vi "CV.vi"(1 "Wait for continue":bool, 2 "Run uninterrupted?":bool, 3 "Device Category IN:":string(combo)="ATLAS18SS" caption="Device Category:", 4 "Batch :":string, 5 "Wafer No.:":string, 6 "DB Serial No.:":string) -> (0 "Done!":bool=TRUE)   [LabVIEW 2018]
doc: "Performs CV measurements according to ATLAS ITk Quality Control Specifications."
uses:
  general_VIs/globals/QC_MeasurementSetup.vi
  general_VIs/globals/QC_RunInformation.vi
  InstrControl/InstrumentSetup.vi
  InstrControl/Switching/Switching.lvclass
  InstrControl/SupplyControl/SupplyControl.lvclass
  InstrControl/LCRControl/LCRControl.lvclass
  InstrControl/ArduinoControl/ArduinoControl.lvclass
  InstrControl/InstrControl.lvclass
panel:
  out "Tab Control 2":enum32{"CV Setup", "CV Scan"}(tab)
  in  "V_depletion limit [V]":dbl=-300.0
  in  "step interval [s] IN":i32=5 caption="step interval [s]"
  in  "step [V] IN":dbl=10.0 caption="step [V]" format="%.1f"
  in  "Final volts [V] IN":dbl=-700.0 caption="Final volts [V]"
  in  "Initial volts [V] IN":dbl caption="Initial volts [V]"
  in  "Current Limit [µA]":dbl=1.0 min=0.0001 format="%.3f"
  in  "Continue":bool
  in  "Quit":bool
  in  "Software current limit?":bool=TRUE
  out "Frequency [Hz] Setup":i32=1000 caption="Frequency [Hz]" format="%#.3p"
  in  "Measurement Configurations":bool
  out "RH":dbl[](array[numeric])=[8.13] caption="RH [%]" format="%#.2f"
  out "step interval [s]":u32=5
  out "step [V]":dbl=10.0 format="%.1f"
  out "Final volts [V]":dbl=-500.0 format="%.1f"
  out "Initial volts [V]":dbl format="%.1f"
  out "Frequency [Hz]":i32=1000 format="%#.3p"
  out "Temp.":dbl[](array[numeric])=[22.58] caption="Temp. [°C]" format="%#.2f"
  out "Volts":dbl[](array[numeric])=[-460.0, -470.0, -480.0, -490.0, -500.0] caption="Volts [V]"
  out "Resistance":dbl[](array[numeric])=[1.56271, 1.56475, 1.51322, 1.51532, 1.51442] caption="Res [kOhm]"
  out "Capacitance":dbl[](array[numeric])=[3119.33, 3118.74, 3118.2400000000002, 3117.68, 3117.2799999999997] caption="Cap [pF]"
  out "Cgraph":cluster{"Initial volts":dbl, dbl, dbl[]}(graph)={"Initial volts"=0.0, 10.0, [5.7235032491421625e-05, 0.003217145788776149, 0.00672998297054733, 0.010666134294020897, 0.014929833398235195, 0.018713223783299704, 0.022188100626603195, 0.025608357885954832, 0.028957991168771992, 0.03227724289159167, 0.03580683190419423, 0.03921028907816598, 0.04253563831220547, 0.045835956575624094, 0.04914718334784051, 0.0524545061658223, 0.055801253982253135, 0.05918861335467005, 0.06262205347418506, 0.06605343343205772, 0.06951342144191594, 0.0730175985670206, 0.07657909511703177, 0.0802264781180157, 0.08403593560473727, 0.08800309677997556, 0.09205485037916886, 0.09598073570407974, 0.09910778032065119, 0.10069600303043066, 0.10132328993192792, 0.1016323293588705, 0.10182246094227795, 0.10197208503414133, 0.10207832275216988, 0.10217166194307145, 0.10225008736408765, 0.1023214020753015, 0.10238361796587031, 0.10244457903006766, 0.10248262532843988, 0.10253579443044537, 0.10258769058231139, 0.10262976192794523, 0.10266988527288097, 0.1027152990629271, 0.10277260288908789, 0.10281149139612399, 0.10284446503963636, 0.10288141435634753, 0.10290781891803549]}
  in  "Scales":T1(ring)
  in  "Cscale":enum16{"1/C^2 [1/nF^2]", "nF", "pF"}(ring)
  out "positive ramp?":bool
  out "Tab Control":enum32{"CV Setup", "CV Scan"}(tab)
  in  "Comments":string caption="Comments:"
  in  "Auto save files":bool=TRUE
  in  "LCR Meter":string(combo)="HP 4284A"
  in  "User:":string(combo)="Vera"
  in  "CV Supply":string(combo)="Keithley 237"
  in  "Hardware Configurations":bool
  in  "Temperature":enum16{"Read Arduino", "Enter manually"}(ring)
  in  "Manufacturer:":string(combo)="Hamamatsu"
  in  "abort":bool
  out "Device Category:":string="ATLAS18SS"
  out "DB Serial No.:":string="20USES50000070"
  out "Current Volts:":dbl format="%.2f"
  in  "quit (no save)":bool
  in  "Quit & Save":bool
  out "Bias On/Off:":bool
  out "STATUS 1":string="Run finished.\nData saved."
  out "Initiated:":string="Thu, Jul 9, 2020"
  out "Wafer:":string="W070"
  out "No of steps":u32=71
  out "Current reading No.":u32=51
  out "Last reading at:":string="2:43:44 PM"
  # "Strip Sensor QC: CV"
  # "University of\nCambridge"
  # "Vertical Scale:"
  # "Measurement Configuration"
  # "CV Scan parameters:"
  # "Last 5 readings:"
  # "n-4"
  # "n-3"
  # "n-2"
  # "n-1"
  # "n"
  # "DUT Description"
  # "Hardware"
  # "DUT & Test Description:"
  # "Current status:"
  # "Rdg No:"
  # "out of"
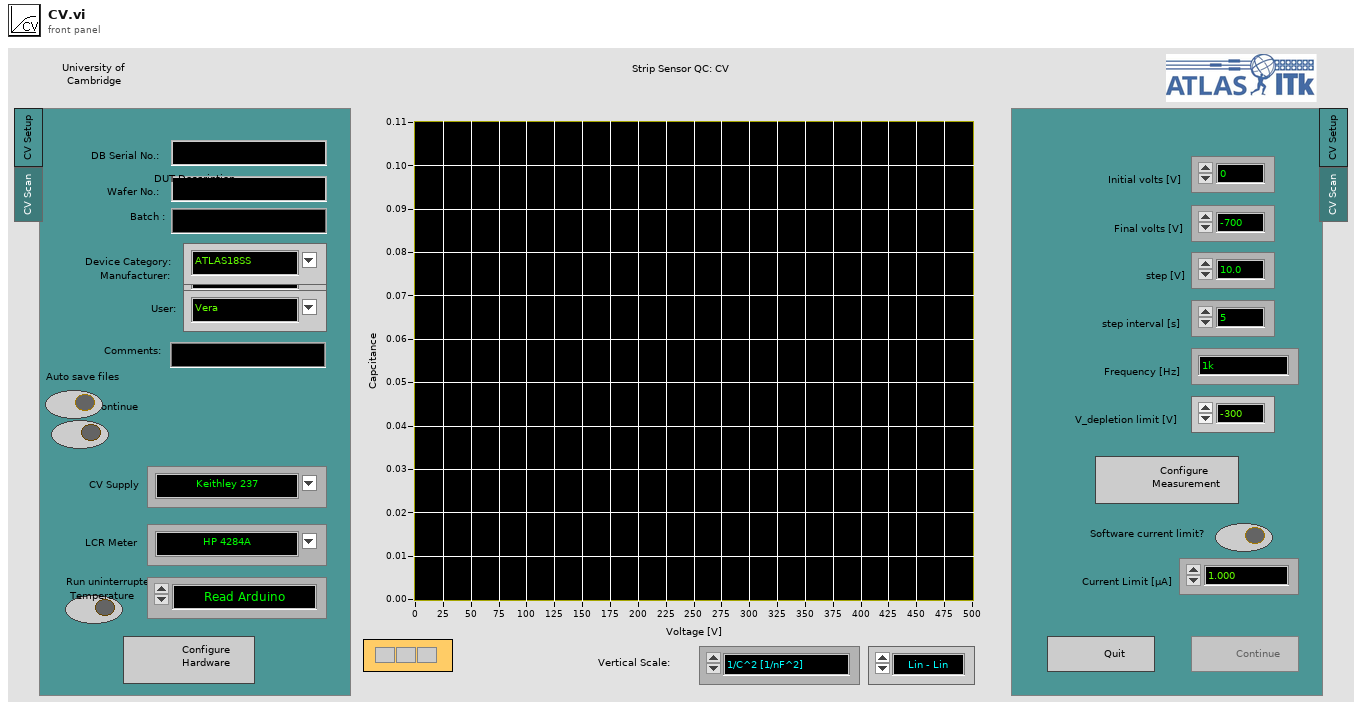
[diagram p1: front panel]
types:
  T1 = enum16{"Lin - Lin", "Log - Lin", "Lin - Log", "Log - log"}
  T2 = enum16{"Supply", "LCR", "Multimeter", "Switching"}
  T3 = enum16{"Reset", "Read Array", "Read Element", "Write Element", "Write Array", "Add Element", "Add Array"}
  T4 = enum16{"Reset", "Ground", "Striptest SMU", "Striptest LCR", "IV", "CV", "Interstrip Cap", "Interstrip Res"}
  T5 = enum32{"IV", "CV", "Stability", "Striptest", "Cis", "Ris", "PTP"}
  T6 = cluster{"Sensor Serial No.:":string, "Wafer:":string, "Batch:":string, "Manufacturer:":string, "Device Category:":string, "Database Serial No.:":string, "Date Initiated:":string, "Time Initiated:":string, "Test":string, "Probeplan used:":string, "End of Run comment:":string, "User:":string, "Vbias SMU":string, "LCR":string, "Test SMU":string, "Test DMM":string, "Comments":string}
  T7 = cluster{"Institute":string, "Manufacturers":string[], "Devices":string[], "Serialnumbers Lookup DB":string, "Data directory":string, "Backup & screenshot directory":string, "List of known users":string[], "Measurement switch not used":bool, "Measurement Switch":string, "DUT Switch":string, "Rseries IV [MOhm]":string, "Rshunt IV [MOhm]":string, "Rseries CV [MOhm]":string, "DC blocking Cap [µF]":string, "Rseries LCR [MOhm]":string, "Rseries stability [MOhm]":string, "Rshunt stability [MOhm]":string, "Rseries striptest bias [MOhm]":string, "Rseries strip pinhole [MOhm]":string}
  T8 = cluster{"Supply":refnum<class "SupplyControl.lvclass">, "LCR":refnum<class "LCRControl.lvclass">, "Arduino":refnum<class "ArduinoControl.lvclass">, "Measurement switch":refnum<class "Switching.lvclass">, "Initial Voltage [V]":dbl, "Final Voltage [V]":dbl, "Step Size [V]":dbl, "Step Interval [s]":i32, "Number Of Steps":u32, "AC frequency [Hz]":i32, "RC Configuration":u16, "AC amplitude [V]":dbl, "Ramp down steps [V]":dbl, "Ramp down Interval [s]":i32, "Set Current Limit?":bool, "Current Limit [µA]":dbl, "Temperature Readout":enum16{"Read Arduino", "Enter manually"}, "Supply Name":string, "LCR Name":string, "V_depletion Limit [V]":dbl, "Measurement switch used?":bool}
  T9 = cluster{"RC Configuration":u16, "AC amplitude [V]":dbl, "Consider OC":bool, "Consider SC":bool, "AC frequency [Hz]":i32, "HP4284A":refnum<class "HP4284A.lvclass">}
  T10 = cluster{"VISA address":refnum<visa-resource-name>, "T sensor":enum16{"SHT", "DS"}, "Arduino":refnum<class "ArduinoControl.lvclass">}
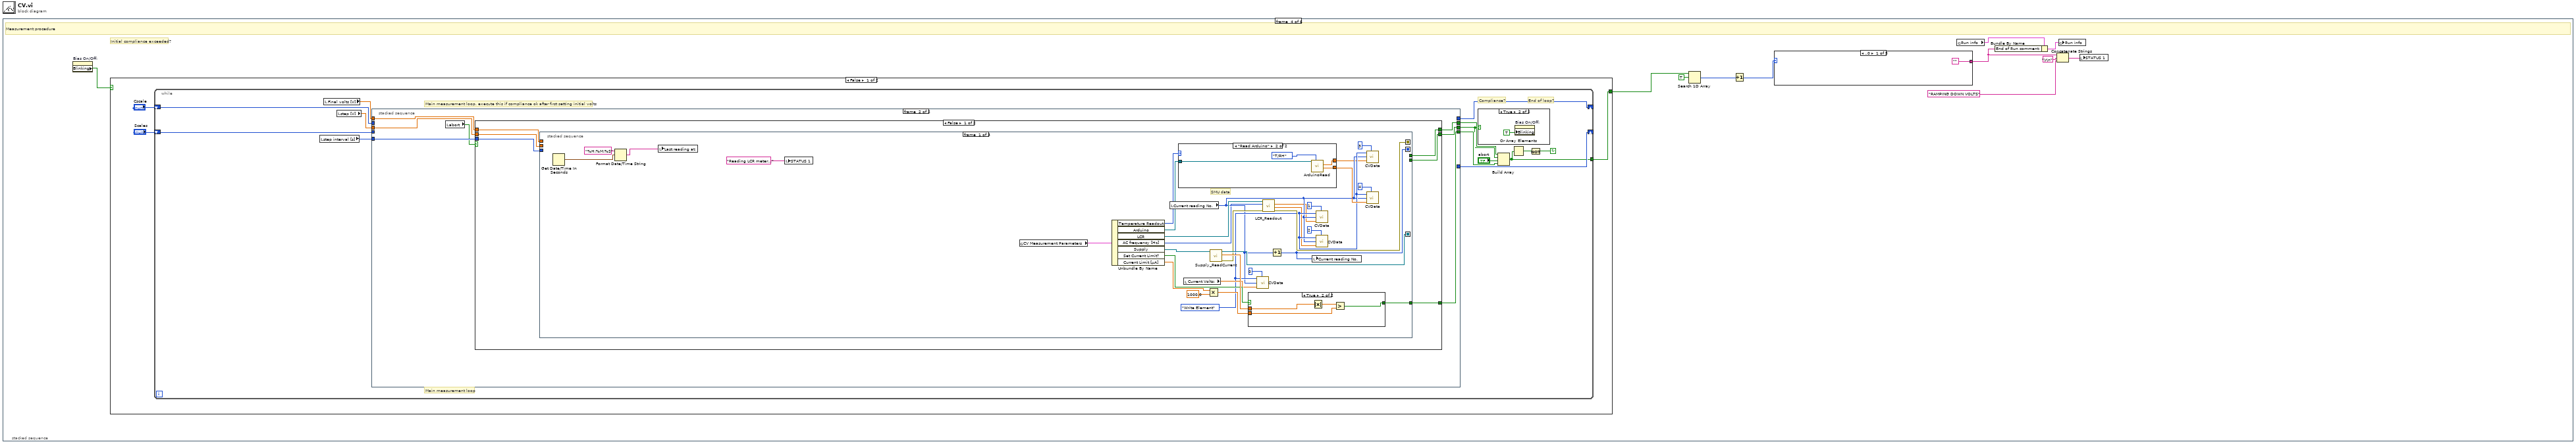
[diagram p0: block diagram]
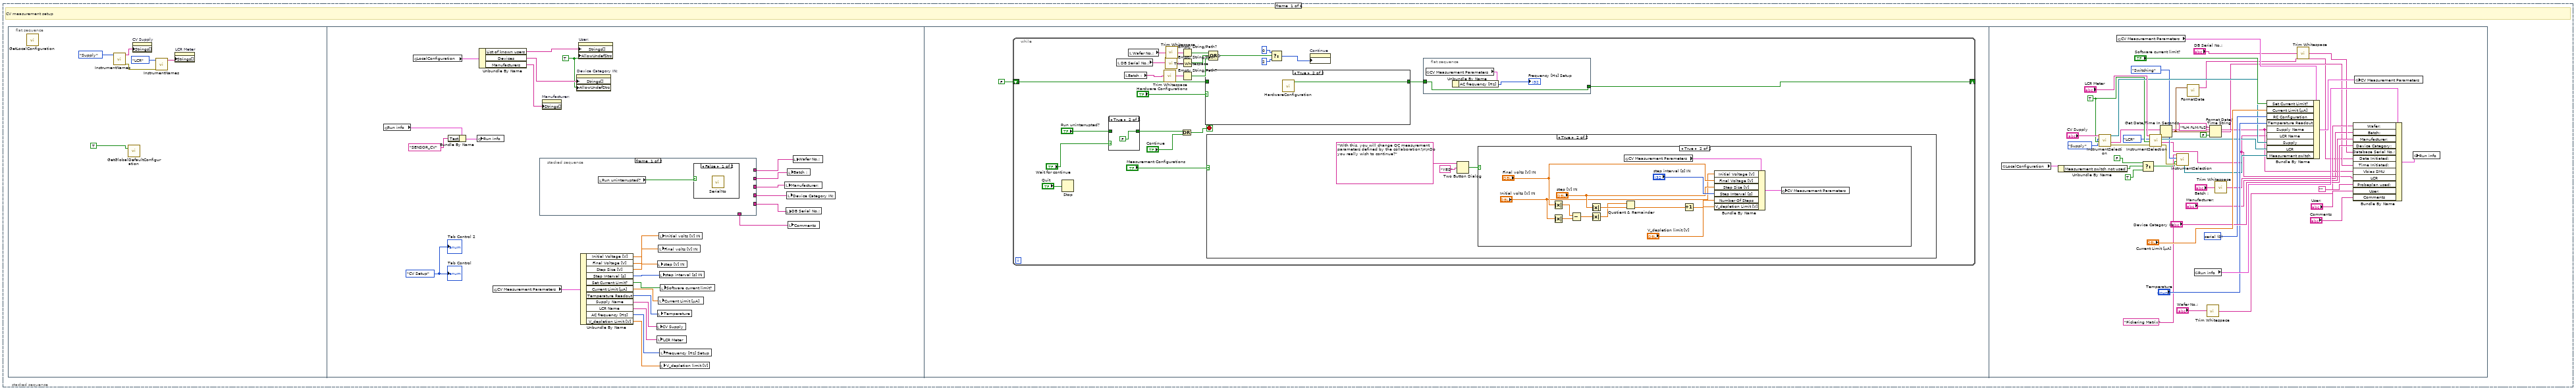
[diagram p2: hidden frame]
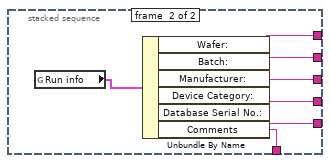
[diagram p4: hidden frame]
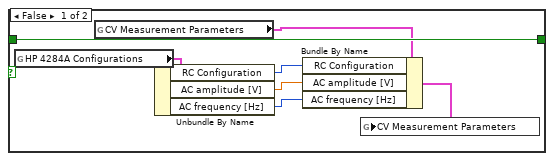
[diagram p6: hidden frame]
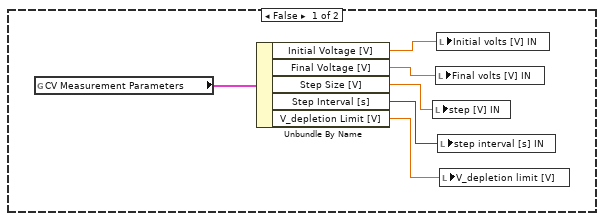
[diagram p8: hidden frame]
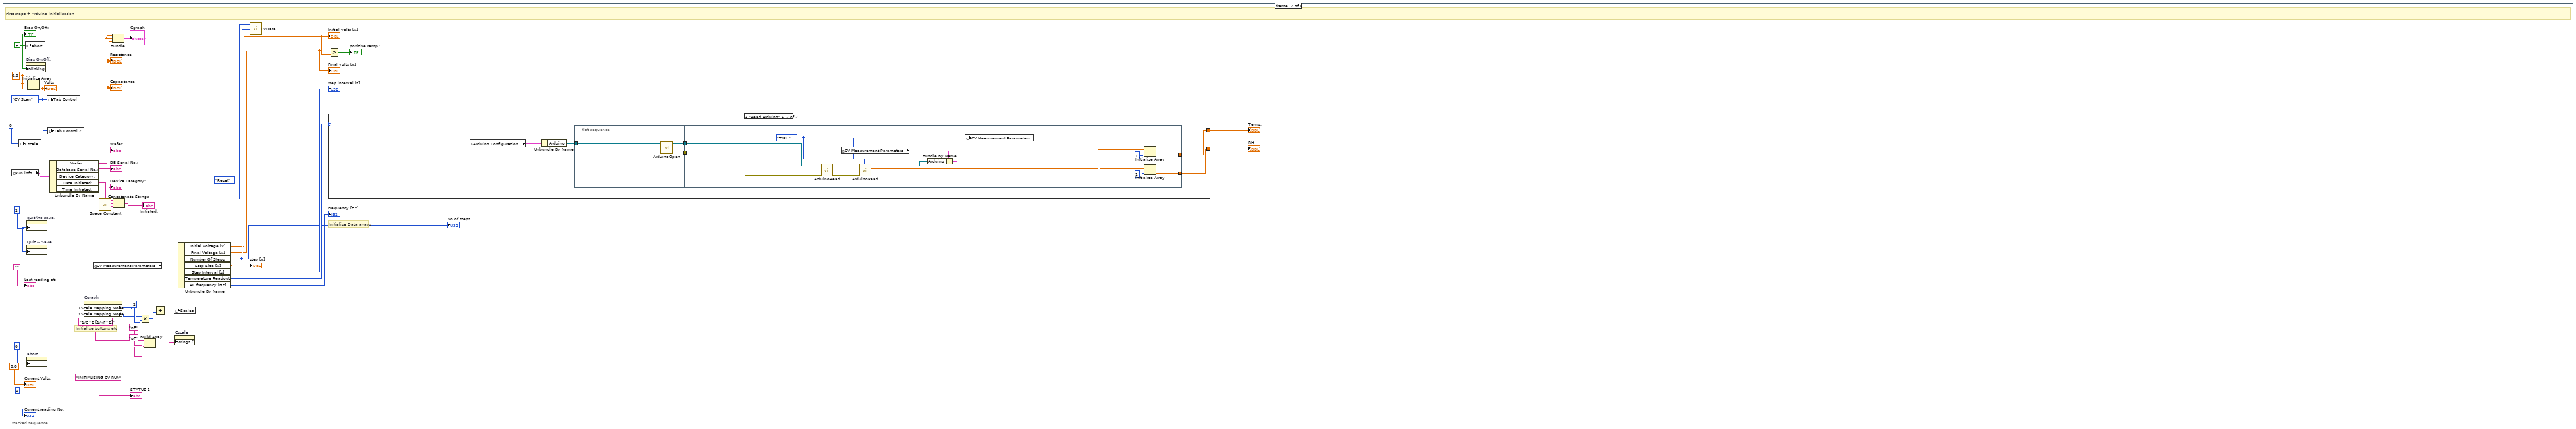
[diagram p9: hidden frame]
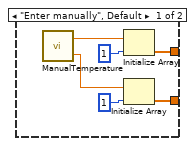
[diagram p10: hidden frame]
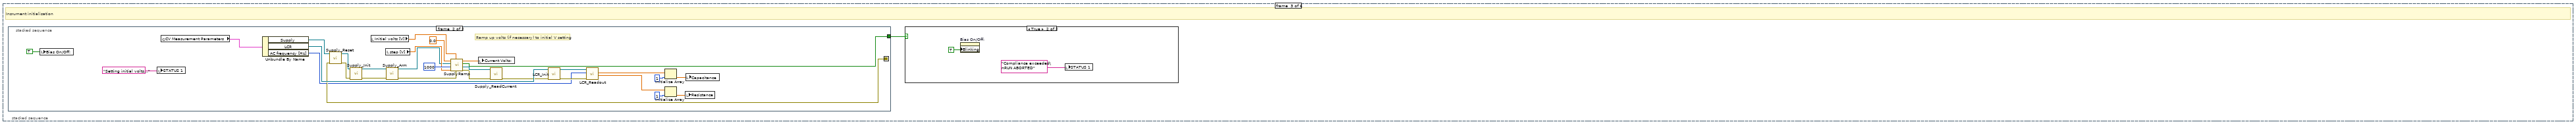
[diagram p11: hidden frame]
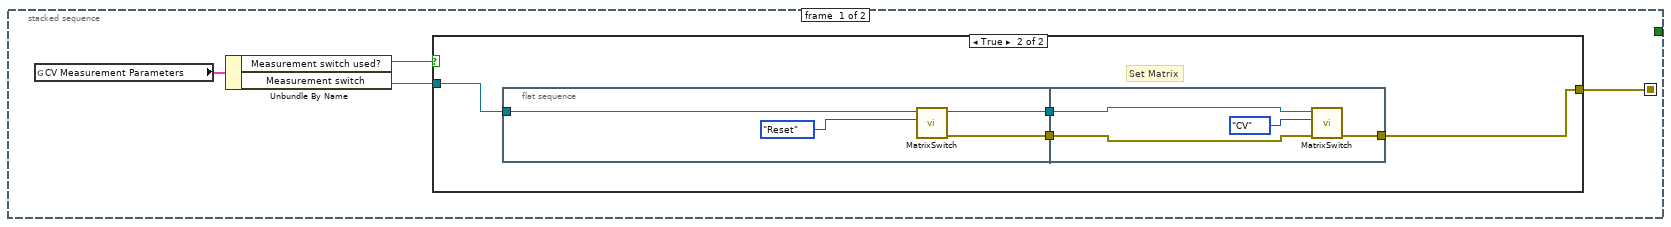
[diagram p12: hidden frame]
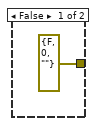
[diagram p13: hidden frame]
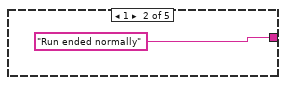
[diagram p15: hidden frame]
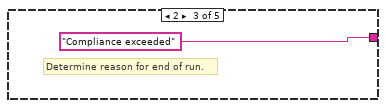
[diagram p16: hidden frame]
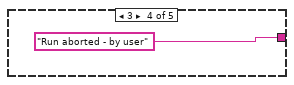
[diagram p17: hidden frame]
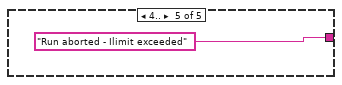
[diagram p18: hidden frame]
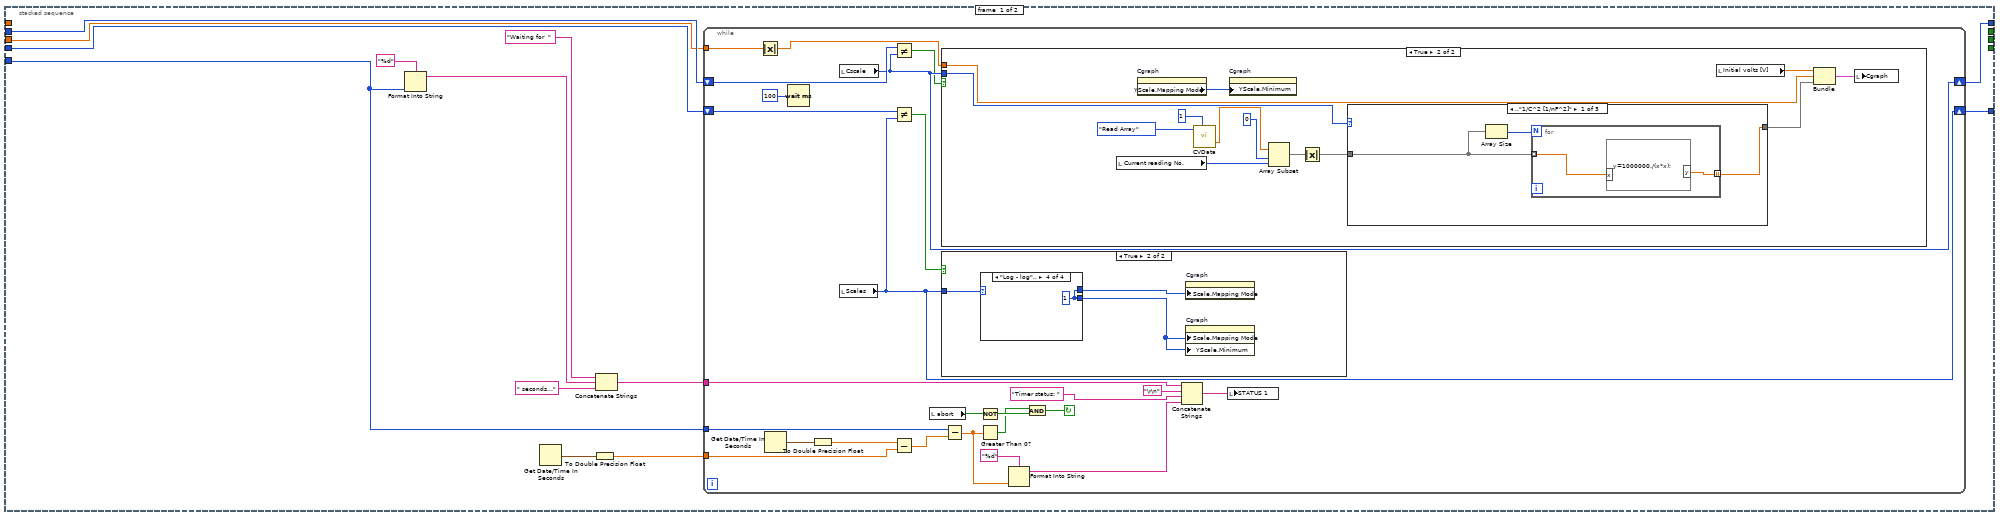
[diagram p19: hidden frame]
diagram:
  n1 = stacked-sequence {
    frame #0 {
      # "CV measurement setup"
      n2 = flat-sequence {
        frame #0 {
          n3 = call "GetLocalConfiguration.vi"() -> ()  [unwired: 3 in, 1 out]
          n4 = call "InstrumentNames.vi"("Instrument type"=T2."Supply") -> ("error out"=w1:errorcluster, "Instrument names"=w3:string[])  [unwired: 9 in]
          n5 = call "GetGlobalDefaultConfiguration.vi"("Read defaults?"=TRUE) -> ()  [unwired: 3 in]
          n6 = property on="CV Supply" class="CmbBox"("Strings[]"=w3) -> ()  [unwired: 2 in, 2 out]
          n7 = call "InstrumentNames.vi"("error in (no error)"=w1, "Instrument type"=T2."LCR") -> ("Instrument names"=w2:string[])  [unwired: 8 in, 1 out]
          n8 = property on="LCR Meter" class="CmbBox"("Strings[]"=w2) -> ()  [unwired: 2 in, 2 out]
        }
        frame #1 {
          w22 = enum32{"CV Setup", "CV Scan"}."CV Setup" ("Tab Control")
          w14 = TRUE
          n9 = global read "QC_RunInformation.vi" "Run info"() -> (w23:T6)
          n10 = global read "QC_RunInformation.vi" "LocalConfiguration"() -> (w28:T7)
          n11 = Bundle By Name(cluster=w23, "Test"="SENSOR_CV") -> (w24:T6)
          n12 = global write "QC_RunInformation.vi" "Run info"(w24) -> ()
          n13 = Unbundle By Name(w28) -> ("List of known users"=w27:string[], "Devices"=w15:string[], "Manufacturers"=w16:string[])
          n14 = global read "QC_MeasurementSetup.vi" "CV Measurement Parameters"() -> (w31:T8)
          n15 = stacked-sequence {
            tunnel: [_ w41] -> w12
            tunnel: [_ w40] -> w11
            tunnel: [_ w39] -> w10
            tunnel: [_ w38] -> w13
            tunnel: [_ w36] -> w9
            tunnel: [_ w35] -> w7
            frame #0 {
              n16 = local read "Run uninterrupted?"() -> (w34:bool)
              n17 = case shown="False" w34 {
                frame False {
                  n18 = call "SerialNo.vi"() -> ()  [unwired: 5 in, 1 out]
                }
                frame True {
                }
              }
            }
            frame #1 {
              n19 = global read "QC_RunInformation.vi" "Run info"() -> (w37:T6)
              n20 = Unbundle By Name(w37) -> ("Wafer:"=w41:string, "Batch:"=w40:string, "Manufacturer:"=w39:string, "Device Category:"=w38:string, "Database Serial No.:"=w36:string, "Comments"=w35:string)
            }
          }
          n21 = property on="Manufacturer:" class="CmbBox"("Strings[]"=w16) -> ()  [unwired: 2 in, 2 out]
          n22 = property on="Device Category IN:" class="CmbBox"("Strings[]"=w15, "AllowUndefStrs"=w14) -> ()  [unwired: 2 in, 2 out]
          n23 = property on="User:" class="CmbBox"("Strings[]"=w27, "AllowUndefStrs"=w14) -> ()  [unwired: 2 in, 2 out]
          n24 = Unbundle By Name(w31) -> ("Initial Voltage [V]"=w18:dbl, "Final Voltage [V]"=w19:dbl, "Step Size [V]"=w20:dbl, "Step Interval [s]"=w21:i32, "Set Current Limit?"=w30:bool, "Current Limit [µA]"=w29:dbl, "Temperature Readout"=w33:enum16{"Read Arduino", "Enter manually"}, "Supply Name"=w32:string, "LCR Name"=w26:string, "AC frequency [Hz]"=w25:i32, "V_depletion Limit [V]"=w17:dbl)
          n25 = local write "CV Supply"(w32) -> ()
          n26 = local write "LCR Meter"(w26) -> ()
          n27 = local write "step [V] IN"(w20) -> ()
          n28 = local write "Temperature"(w33) -> ()
          n29 = local write "Final volts [V] IN"(w19) -> ()
          n30 = local write "Current Limit [µA]"(w29) -> ()
          n31 = local write "Initial volts [V] IN"(w18) -> ()
          n32 = local write "step interval [s] IN"(w21) -> ()
          n33 = local write "Frequency [Hz] Setup"(w25) -> ()
          n34 = local write "V_depletion limit [V]"(w17) -> ()
          n35 = local write "Software current limit?"(w30) -> ()
          n36 = local write "Manufacturer:"(w10) -> ()
          n37 = local write "DB Serial No.:"(w9) -> ()
          n38 = local write "Device Category IN:"(w13) -> ()
          n39 = local write "Batch :"(w11) -> ()
          n40 = local write "Comments"(w7) -> ()
          n41 = local write "Wafer No.:"(w12) -> ()
          "Tab Control" <- w22
          "Tab Control 2" <- w22
        }
        frame #2 {
          n42 = while {
            shift-right: [w43] -> _
            shift-left: FALSE -> [w55]
            stop <- w57 stop-if-true
            n43 = Stop(stop? (T)="Quit") -> ()
            n44 = case shown="True" "Wait for continue" {
              tunnel: "Run uninterrupted?" -> [w70 _]
              tunnel: [w70 FALSE] -> w51
              frame False {
              }
              frame True {
              }
            }
            n45 = local read "DB Serial No.:"() -> (w48:string)
            n46 = local read "Batch :"() -> (w46:string)
            n47 = local read "Wafer No.:"() -> (w49:string)
            n48 = call <vilib>:"Trim Whitespace.vi"("string"=w46) -> ("trimmed string"=w45:string)  [unwired: 1 in]
            n49 = call <vilib>:"Trim Whitespace.vi"("string"=w48) -> ("trimmed string"=w47:string)  [unwired: 1 in]
            n50 = call <vilib>:"Trim Whitespace.vi"("string"=w49) -> ("trimmed string"=w50:string)  [unwired: 1 in]
            n51 = Or(x=w51, y="Continue") -> (x .or. y?=w57:bool)
            n52 = Empty String/Path?(string/path=w50) -> (empty?=w64:bool)
            n53 = Empty String/Path?(string/path=w47) -> (empty?=w65:bool)
            n54 = Empty String/Path?(string/path=w45) -> (empty?=w59:bool)
            n55 = case shown="True" "Hardware Configurations" {
              tunnel: [w78 w79] -> w44
              tunnel: w55 -> [w78 _]
              frame False {
                n56 = global read "InstrumentSetup.vi" "HP 4284A Configurations"() -> (w77:T9)
                n57 = global read "QC_MeasurementSetup.vi" "CV Measurement Parameters"() -> (w76:T8)
                n58 = Unbundle By Name(w77) -> ("RC Configuration"=w75:u16, "AC amplitude [V]"=w74:dbl, "AC frequency [Hz]"=w73:i32)
                n59 = Bundle By Name(cluster=w76, "RC Configuration"=w75, "AC amplitude [V]"=w74, "AC frequency [Hz]"=w73) -> (w72:T8)
                n60 = global write "QC_MeasurementSetup.vi" "CV Measurement Parameters"(w72) -> ()
              }
              frame True {
                n61 = call "HardwareConfiguration.vi"() -> ("configured?"=w79:bool)  [unwired: 11 in]
              }
            }
            n62 = case shown="True" "Measurement Configurations" {
              frame False {
              }
              frame True {
                n63 = Two Button Dialog(message="With this, you will change QC measurement parameters defined by the collaboration!\n\nDo you really wish to continue?", 2:"YES") -> (T button?=w80:bool)  [unwired: 1 in]
                n64 = case shown="True" w80 {
                  frame False {
                    n65 = global read "QC_MeasurementSetup.vi" "CV Measurement Parameters"() -> (w88:T8)
                    n66 = Unbundle By Name(w88) -> ("Initial Voltage [V]"=w85:dbl, "Final Voltage [V]"=w84:dbl, "Step Size [V]"=w86:dbl, "Step Interval [s]"=w87:i32, "V_depletion Limit [V]"=w83:dbl)
                    n67 = local write "step [V] IN"(w86) -> ()
                    n68 = local write "Final volts [V] IN"(w84) -> ()
                    n69 = local write "Initial volts [V] IN"(w85) -> ()
                    n70 = local write "step interval [s] IN"(w87) -> ()
                    n71 = local write "V_depletion limit [V]"(w83) -> ()
                  }
                  frame True {
                    n72 = Absolute Value(x="Final volts [V] IN") -> (abs(x)=w94:dbl)
                    n73 = Absolute Value(x="Initial volts [V] IN") -> (abs(x)=w95:dbl)
                    n74 = Subtract(x=w94, y=w95) -> (x-y=w98:dbl)
                    n75 = Absolute Value(x="step [V] IN") -> (abs(x)=w97:dbl)
                    n76 = Absolute Value(x=w98) -> (abs(x)=w96:dbl)
                    n77 = global read "QC_MeasurementSetup.vi" "CV Measurement Parameters"() -> (w102:T8)
                    n78 = Quotient & Remainder(x=w96, y=w97) -> (floor(x/y)=w93:dbl)  [unwired: 1 out]
                    n79 = Increment(x=w93) -> (x+1=w92:dbl)
                    n80 = Bundle By Name(cluster=w102, "Initial Voltage [V]"="Initial volts [V] IN", "Final Voltage [V]"="Final volts [V] IN", "Step Size [V]"="step [V] IN", "Step Interval [s]"="step interval [s] IN", "Number Of Steps"=w92, "V_depletion Limit [V]"="V_depletion limit [V]") -> (w101:T8)
                    n81 = global write "QC_MeasurementSetup.vi" "CV Measurement Parameters"(w101) -> ()
                  }
                }
              }
            }
            n82 = Compound Arithmetic op=OR(w64, w65, w59) -> (invert w63:bool)
            n83 = Select(t=0, s=w63, f=2) -> (s? t:f=w60:i32)
            n84 = property on="Continue" class="Bool"("DisabledEnum"=w60) -> ()  [unwired: 2 in, 2 out]
            n85 = flat-sequence {
              tunnel: w44 -> [w67]
              tunnel: [w67] -> w43
              frame #0 {
                n86 = global read "QC_MeasurementSetup.vi" "CV Measurement Parameters"() -> (w69:T8)
                n87 = Unbundle By Name(w69) -> ("AC frequency [Hz]"=→"Frequency [Hz] Setup":i32)
              }
            }
          }
        }
        frame #3 {
          w126 = TRUE
          w136 = u16 0 items=["serial", "parallel"] ("RC Configuration")
          n88 = global read "QC_RunInformation.vi" "LocalConfiguration"() -> (w121:T7)
          n89 = Unbundle By Name(w121) -> ("Measurement switch not used"=w120:bool)
          n90 = call "InstrumentSelection.vi"("Verify GPIB address"=w126, "Instrument type"=T2."Supply", "Instrument name IN"="CV Supply") -> ("error out"=w132:errorcluster, "Instrument name OUT"=w116:string, "Supply"=w131:refnum<class "SupplyControl.lvclass">)  [unwired: 3 in, 3 out]
          n91 = global read "QC_MeasurementSetup.vi" "CV Measurement Parameters"() -> (w144:T8)
          n92 = Select(t=FALSE, s=w120, f=TRUE) -> (s? t:f=w117:bool)
          n93 = call "InstrumentSelection.vi"("error in (no error)"=w132, "Verify GPIB address"=w126, "Instrument type"=T2."LCR", "Instrument name IN"="LCR Meter") -> ("error out"=w128:errorcluster, "Instrument name OUT"=w115:string, "LCR"=w130:refnum<class "LCRControl.lvclass">)  [unwired: 2 in, 3 out]
          n94 = Get Date/Time In Seconds() -> (seconds since 1Jan1904=w104:timestamp)
          n95 = call "InstrumentSelection.vi"("error in (no error)"=w128, "Verify GPIB address"=w117, "Instrument type"=T2."Switching", "Instrument name IN"="Pickering Matrix") -> ("Switching"=w127:refnum<class "Switching.lvclass">)  [unwired: 2 in, 5 out]
          n96 = call "FormatDate.vi"("time stamp"=w104) -> ("Date"=w103:string)  [unwired: 1 in, 1 out]
          n97 = global read "QC_RunInformation.vi" "Run info"() -> (w141:T6)
          n98 = call <vilib>:"Trim Whitespace.vi"("string"="Wafer No.:") -> ("trimmed string"=w108:string)  [unwired: 1 in]
          n99 = Format Date/Time String(time format string (%c)="%H:%M:%S", seconds (now)=w104, UTC format=FALSE) -> (date/time string=w105:string)
          n100 = call <vilib>:"Trim Whitespace.vi"("string"="Batch :") -> ("trimmed string"=w110:string)  [unwired: 1 in]
          n101 = Bundle By Name(cluster=w144, "Set Current Limit?"="Software current limit?", "Current Limit [µA]"="Current Limit [µA]", "RC Configuration"=w136, "Temperature Readout"="Temperature", "Supply Name"=w116, "LCR Name"=w115, "Supply"=w131, "LCR"=w130, "Measurement switch"=w127) -> (w145:T8)
          n102 = call <vilib>:"Trim Whitespace.vi"("string"="DB Serial No.:") -> ("trimmed string"=w112:string)  [unwired: 1 in]
          n103 = Bundle By Name(cluster=w141, "Wafer:"=w108, "Batch:"=w110, "Manufacturer:"="Manufacturer:", "Device Category:"="Device Category IN:", "Database Serial No.:"=w112, "Date Initiated:"=w103, "Time Initiated:"=w105, "Vbias SMU"=w116, "LCR"=w115, "Probeplan used:"="", "User:"="User:", "Comments"="Comments") -> (w140:T6)
          n104 = global write "QC_MeasurementSetup.vi" "CV Measurement Parameters"(w145) -> ()
          n105 = global write "QC_RunInformation.vi" "Run info"(w140) -> ()
        }
      }
    }
    frame #1 {
      w151 = enum32{"CV Setup", "CV Scan"}."CV Scan" ("Tab Control")
      w168 = 2
      w175 = 0.0
      w167 = FALSE ("Visible")
      # "Initialise buttons etc"
      # "Initialise Data arrays"
      # "First steps + Arduino initialisation"
      n106 = global read "QC_RunInformation.vi" "Run info"() -> (w185:T6)
      n107 = local write "Cscale"(u16 0 ("Scale")) -> ()
      n108 = local write "abort"(w167) -> ()
      n109 = property on="Bias On/Off:" class="Bool (strict)"("Blinking"=w167) -> ()  [unwired: 2 in, 2 out]
      n110 = property on="quit (no save)" class="Bool"("DisabledEnum"=w168) -> ()  [unwired: 2 in, 2 out]
      n111 = property on="Quit & Save" class="Bool"("DisabledEnum"=w168) -> ()  [unwired: 2 in, 2 out]
      n112 = property on="abort" class="Bool (strict)"("DisabledEnum"=0) -> ()  [unwired: 2 in, 2 out]
      n113 = Initialize Array(w175, w175) -> (w153:dbl[])
      "Volts" <- w153
      "Capacitance" <- w153
      "Resistance" <- w153
      n114 = local write "Tab Control"(w151) -> ()
      n115 = local write "Tab Control 2"(w151) -> ()
      n116 = Unbundle By Name(w185) -> ("Wafer:"=→"Wafer:":string, "Database Serial No.:"=→"DB Serial No.:":string, "Device Category:"=→"Device Category:":string, "Date Initiated:"=w149:string, "Time Initiated:"=w147:string)
      n117 = property on="Cgraph" class="WFGraph (strict)"() -> ("XScale.Mapping Mode"=w160:u8, "YScale.Mapping Mode"=w159:u8)  [unwired: 2 in, 2 out]
      n118 = global read "QC_MeasurementSetup.vi" "CV Measurement Parameters"() -> (w156:T8)
      n119 = call <vilib>:"Space Constant.vi"() -> ("String"=w148:string)
      n120 = Bundle(w175, w175, w153) -> (→"Cgraph":cluster{dbl, dbl, dbl[]})  [unwired: 1 in]
      n121 = Concatenate Strings(w149, w148, w147) -> (→"Initiated:":string)
      n122 = Multiply(x=w159, y=2) -> (x*y=w162:i32)
      n123 = Build Array("1/C^2 [1/nF^2]", "nF", "pF") -> (w182:string[])
      n124 = Add(x=w160, y=w162) -> (x+y=w158:i32)
      n125 = local write "Scales"(w158) -> ()
      n126 = property on="Cscale" class="Enum (strict)"("Strings []"=w182) -> ()  [unwired: 2 in, 2 out]
      n127 = Unbundle By Name(w156) -> ("Initial Voltage [V]"=w166:dbl, "Final Voltage [V]"=w165:dbl, "Number Of Steps"=w176:u32, "Step Size [V]"=→"step [V]":dbl, "Step Interval [s]"=→"step interval [s]":i32, "Temperature Readout"=w169:enum16{"Read Arduino", "Enter manually"}, "AC frequency [Hz]"=→"Frequency [Hz]":i32)
      "No of steps" <- w176
      "Initial volts [V]" <- w166
      "Final volts [V]" <- w165
      n128 = call "CVData.vi"("Action"=T3."Reset", "Array Size / Index"=w176) -> ()  [unwired: 3 in, 2 out]
      n129 = case shown="\"Read Arduino\"" w169 {
        tunnel: [w191 w198] -> w172
        tunnel: [w188 w197] -> w157
        frame "Enter manually", Default {
          n130 = call "ManualTemperature.vi"() -> ("Humidity [%] out"=w187:dbl, "Temperature [°C] out"=w192:dbl)
          n131 = Initialize Array(w192, 1) -> (w191:dbl[])
          n132 = Initialize Array(w187, 1) -> (w188:dbl[])
        }
        frame "Read Arduino" {
          n133 = global read "InstrumentSetup.vi" "Arduino Configuration"() -> (w194:T10)
          n134 = Unbundle By Name(w194) -> ("Arduino"=w193:refnum<class "ArduinoControl.lvclass">)
          n135 = flat-sequence {
            tunnel: [w199] -> w196
            tunnel: [w201] -> w195
            tunnel: w193 -> [w200]
            tunnel: [w215] -> w198
            tunnel: [w212] -> w197
            tunnel: w196 -> [w204]
            tunnel: w195 -> [w205]
            frame #0 {
              n136 = call "ArduinoOpen.vi"("ArduinoControl in"=w200) -> ("error out"=w201:errorcluster, "ArduinoControl out"=w199:refnum<class "ArduinoControl.lvclass">)  [unwired: 9 in]
            }
            frame #1 {
              w206 = enum16{"T/RH", "Interlock", "Edgesense"}."T/RH" ("Arduino function")
              n137 = call "ArduinoRead.vi"("Arduino function"=w206, "error in (no error)"=w205, "ArduinoControl in"=w204) -> ("error out"=w202:errorcluster, "ArduinoControl out"=w203:refnum<class "ArduinoControl.lvclass">)  [unwired: 3 in, 4 out]
              n138 = global read "QC_MeasurementSetup.vi" "CV Measurement Parameters"() -> (w208:T8)
              n139 = call "ArduinoRead.vi"("Arduino function"=w206, "error in (no error)"=w202, "ArduinoControl in"=w203) -> ("rel. Humidity [%]"=w210:dbl, "Temperature [°C]"=w211:dbl, "ArduinoControl out"=w209:refnum<class "ArduinoControl.lvclass">)  [unwired: 3 in, 3 out]
              n140 = Bundle By Name(cluster=w208, "Arduino"=w209) -> (w207:T8)
              n141 = global write "QC_MeasurementSetup.vi" "CV Measurement Parameters"(w207) -> ()
              n142 = Initialize Array(w211, 1) -> (w215:dbl[])
              n143 = Initialize Array(w210, 1) -> (w212:dbl[])
            }
          }
        }
      }
      "Temp." <- w172
      "RH" <- w157
      n144 = Greater?(x=w165, y=w166) -> (0:→"positive ramp?":bool)
      "STATUS 1" <- "INITIALISING CV RUN"
      "Bias On/Off:" <- w167
      "Last reading at:" <- ""
      "Current reading No." <- u32 0 ("Current reading No.")
      "Current Volts:" <- 0.0 ("Current Volts:")
    }
    frame #2 {
      # "Insrument initialisation"
      n145 = stacked-sequence {
        seq-local: [w218 _] -> [_ w241]
        tunnel: [_ w245] -> w216
        frame #0 {
          n146 = global read "QC_MeasurementSetup.vi" "CV Measurement Parameters"() -> (w217:T8)
          n147 = Unbundle By Name(w217) -> ("Measurement switch used?"=w220:bool, "Measurement switch"=w219:refnum<class "Switching.lvclass">)
          n148 = case shown="True" w220 {
            tunnel: w219 -> [_ w222]
            tunnel: [errorcluster {"status"=FALSE, "code"=0, "source"=""} ("error constant") w223] -> w218
            frame False {
            }
            frame True {
              # "Set Matrix"
              n149 = flat-sequence {
                tunnel: [w229] -> w225
                tunnel: [w228] -> w224
                tunnel: w222 -> [w226]
                tunnel: w225 -> [w233]
                tunnel: w224 -> [w232]
                tunnel: [w231] -> w223
                frame #0 {
                  n150 = call-dynamic "MatrixSwitch.vi"("Action"=T4."Reset", "Switching in"=w226) -> ("error out"=w229:errorcluster, "Switching out"=w228:refnum<class "Switching.lvclass">)  [unwired: 7 in, 1 out]
                }
                frame #1 {
                  n151 = call-dynamic "MatrixSwitch.vi"("error in (no error)"=w233, "Action"=T4."CV", "Switching in"=w232) -> ("error out"=w231:errorcluster)  [unwired: 6 in, 2 out]
                }
              }
            }
          }
        }
        frame #1 {
          # "Ramp up volts (if necessary) to initial V setting"
          n152 = local write "Bias On/Off:"(TRUE ("Compliance?")) -> ()
          n153 = local write "STATUS 1"("Setting initial volts..." ("STATUS 1")) -> ()
          n154 = global read "QC_MeasurementSetup.vi" "CV Measurement Parameters"() -> (w259:T8)
          n155 = Unbundle By Name(w259) -> ("Supply"=w256:refnum<class "SupplyControl.lvclass">, "LCR"=w255:refnum<class "LCRControl.lvclass">, "AC frequency [Hz]"=w234:i32)
          n156 = call-dynamic "Supply_Reset.vi"("error in (no error)"=w241, "SupplyControl in"=w256) -> ("error out"=w261:errorcluster, "SupplyControl out"=w263:refnum<class "SupplyControl.lvclass">)  [unwired: 8 in]
          n157 = call-dynamic "Supply_Init.vi"("error in (no error)"=w261, "SupplyControl in"=w263) -> ("error out"=w260:errorcluster, "SupplyControl out"=w262:refnum<class "SupplyControl.lvclass">)  [unwired: 8 in]
          n158 = local read "Initial volts [V]"() -> (w248:dbl)
          n159 = local read "step [V]"() -> (w249:dbl)
          n160 = call-dynamic "Supply_Arm.vi"("error in (no error)"=w260, "SupplyControl in"=w262) -> ("error out"=w243:errorcluster, "SupplyControl out"=w244:refnum<class "SupplyControl.lvclass">)  [unwired: 8 in]
          n161 = call "SupplyRamp.vi"("error in"=w243, "Requested Voltage"=w248, "Step Size"=w249, "Step Delay"=1000, "Supply IN"=w244, "Starting Voltage"=0.0) -> ("error out"=w246:errorcluster, "Supply OUT"=w247:refnum<class "SupplyControl.lvclass">, "Compliance exceeded"=w245:bool, "Current Voltage"=w252:dbl)  [unwired: 2 in]
          n162 = local write "Current Volts:"(w252) -> ()
          n163 = call-dynamic "Supply_ReadCurrent.vi"("error in (no error)"=w246, "SupplyControl in"=w247) -> ("error out"=w242:errorcluster)  [unwired: 7 in, 2 out]
          n164 = call-dynamic "LCR_Init.vi"("error in (no error)"=w242, "LCRControl in"=w255) -> ("error out"=w239:errorcluster, "LCRControl out"=w240:refnum<class "LCRControl.lvclass">)  [unwired: 8 in]
          n165 = call-dynamic "LCR_Readout.vi"("error in (no error)"=w239, "Frequency in Hz"=w234, "LCRControl in"=w240) -> ("Resistance in Ohm"=w236:dbl, "Capacitance in pF"=w238:dbl)  [unwired: 5 in, 2 out]
          n166 = Initialize Array(w238, 1) -> (w253:dbl[])
          n167 = Initialize Array(w236, 1) -> (w235:dbl[])
          n168 = local write "Resistance"(w235) -> ()
          n169 = local write "Capacitance"(w253) -> ()
        }
      }
      n170 = case shown="True" w216 {
        frame False {
        }
        frame True {
          n171 = property on="Bias On/Off:" class="Bool (strict)"("Blinking"=TRUE) -> ()  [unwired: 2 in, 2 out]
          n172 = local write "STATUS 1"("Compliance exceeded\nRUN ABORTED") -> ()
        }
      }
    }
    frame #3 {
      # "Initial compliance exceeded?"
      # "Measurement procedure"
      n173 = property on="Bias On/Off:" class="Bool (strict)"() -> ("Blinking"=w276:bool)  [unwired: 2 in, 2 out]
      n174 = case shown="False" w276 {
        tunnel: [w284 w532] -> w275
        frame False {
          n175 = while {
            shift-left: "Cscale" -> [w294]
            shift-right: [w293] -> _
            shift-left: "Scales" -> [w295]
            shift-right: [w296] -> _
            tunnel: [w292] -> w284
            stop <- w297 continue-if-true
            # "Main measurement loop"
            # "End of loop?"
            # "Compliance?"
            # "Main measurement loop. execute this if compliance ok after first setting initial volts"
            n176 = local read "step interval [s]"() -> (w289:u32)
            n177 = local read "Final volts [V]"() -> (w290:dbl)
            n178 = local read "step [V]"() -> (w291:dbl)
            n179 = stacked-sequence {
              tunnel: [w311 _] -> w296
              tunnel: w291 -> [w308 w374]
              tunnel: [_ w373] -> w286
              tunnel: w290 -> [_ w372]
              tunnel: w289 -> [w299 w371]
              tunnel: [_ w370] -> w288
              tunnel: w295 -> [w310 _]
              tunnel: w294 -> [w309 _]
              tunnel: [w307 _] -> w293
              tunnel: [_ w368] -> w287
              frame #0 {
                n180 = Format Into String(format string="%d", w299) -> (resulting string=w304:string)  [unwired: 2 in, 1 out]
                n181 = Get Date/Time In Seconds() -> (seconds since 1Jan1904=w301:timestamp)
                n182 = To Double Precision Float(number=w301) -> (double precision float=w302:dbl)
                n183 = Concatenate Strings("Waiting for  ", w304, " seconds...") -> (w300:string)
                n184 = while {
                  tunnel: w308 -> [w320]
                  shift-left: w309 -> [w324]
                  shift-right: [w317] -> w307
                  shift-left: w310 -> [w325]
                  shift-right: [w326] -> w311
                  tunnel: w300 -> [w318]
                  tunnel: w299 -> [w330]
                  tunnel: w302 -> [w331]
                  stop <- w332 continue-if-true
                  n185 = Absolute Value(x=w320) -> (abs(x)=w319:dbl)
                  n186 = Get Date/Time In Seconds() -> (seconds since 1Jan1904=w316:timestamp)
                  n187 = Wait (ms)(milliseconds to wait=u32 100) -> ()  [unwired: 1 out]
                  n188 = To Double Precision Float(number=w316) -> (double precision float=w336:dbl)
                  n189 = local read "Cscale"() -> (w317:enum16{"1/C^2 [1/nF^2]", "nF", "pF"})
                  n190 = local read "Scales"() -> (w326:T1)
                  n191 = Not Equal?(x=w324, y=w317) -> (x != y?=w315:bool)
                  n192 = Not Equal?(x=w325, y=w326) -> (x != y?=w327:bool)
                  n193 = Subtract(x=w336, y=w331) -> (x-y=w313:dbl)
                  n194 = local read "abort"() -> (w329:bool)
                  n195 = case shown="True" w315 {
                    tunnel: w319 -> [_ w348]
                    tunnel: w317 -> [_ w341]
                    frame False {
                    }
                    frame True {
                      n196 = local read "Current reading No."() -> (w346:u32)
                      n197 = property on="Cgraph" class="WFGraph (strict)"() -> ("YScale.Mapping Mode"=w343:u8)  [unwired: 2 in, 2 out]
                      n198 = call "CVData.vi"("Action"=T3."Read Array", "Array No."=u32 1 ("Action")) -> ("Array OUT"=w337:dbl[])  [unwired: 3 in, 1 out]
                      n199 = property on="Cgraph" class="WFGraph (strict)"("YScale.Minimum"=w343) -> ()  [unwired: 2 in, 2 out]
                      n200 = Array Subset(array=w337, index=0, length=w346) -> (w344:dbl[])
                      n201 = Absolute Value(x=w344) -> (abs(x)=w342:dbl[])
                      n202 = case shown="..\"1/C^2 [1/nF^2]\"" w341 {
                        tunnel: [w352 w355 w358] -> w340
                        tunnel: w342 -> [w350 w357 w358]
                        frame .."1/C^2 [1/nF^2]" {
                          n203 = Array Size(array=w350) -> (size(s)=w351:i32)
                          n204 = for {
                            N: w351 -> [_]
                            tunnel: w350 -> [w354] mode=indexing
                            tunnel: [w353] -> w352 mode=indexing
                            n205 = formula code="y=1000000./(x*x);"("x"=w354) -> ("y"=w353:dbl)
                          }
                        }
                        frame "nF" {
                          n206 = Divide(x=w357, y=1000.0) -> (x/y=w355:dbl[])
                        }
                        frame "pF".. {
                        }
                      }
                      n207 = local read "Initial volts [V]"() -> (w347:dbl)
                      n208 = Bundle("Initial volts [V]"=w347, w348, w340) -> (w345:cluster{"Initial volts [V]":dbl, dbl, dbl[]})  [unwired: 1 in]
                      n209 = local write "Cgraph"(w345) -> ()
                    }
                  }
                  n210 = case shown="True" w327 {
                    tunnel: w326 -> [_ w361]
                    frame False {
                    }
                    frame True {
                      n211 = case shown="\"Log - log\".." w361 {
                        tunnel: [w362 1 0 w367] -> w360
                        tunnel: [w362 0 1 w367] -> w359
                        frame .."Lin - Lin" {
                          w362 = 0
                        }
                        frame "Log - Lin" {
                        }
                        frame "Lin - Log" {
                        }
                        frame "Log - log".. {
                          w367 = 1
                        }
                      }
                      n212 = property on="Cgraph" class="WFGraph (strict)"("X Scale.Mapping Mode"=w360) -> ()  [unwired: 2 in, 2 out]
                      n213 = property on="Cgraph" class="WFGraph (strict)"("Y Scale.Mapping Mode"=w359, "YScale.Minimum"=w359) -> ()  [unwired: 2 in, 2 out]
                    }
                  }
                  n214 = Subtract(x=w330, y=w313) -> (x-y=w312:dbl)
                  n215 = Not(x=w329) -> (.not. x?=w335:bool)
                  n216 = Greater Than 0?(x=w312) -> (x > 0?=w314:bool)
                  n217 = Format Into String(format string="%d", w312) -> (resulting string=w334:string)  [unwired: 2 in, 1 out]
                  n218 = And(x=w314, y=w335) -> (x .and. y?=w332:bool)
                  n219 = Concatenate Strings(w318, "\r\n", "Timer status: ", w334) -> (w328:string)
                  n220 = local write "STATUS 1"(w328) -> ()
                }
              }
              frame #1 {
                n221 = local read "abort"() -> (w369:bool)
                n222 = case shown="False" w369 {
                  tunnel: [w380 w529] -> w370
                  tunnel: w371 -> [w379 _]
                  tunnel: w372 -> [w378 _]
                  tunnel: [w376 w529] -> w373
                  tunnel: w374 -> [w377 _]
                  tunnel: [w375 w529] -> w368
                  frame False {
                    n223 = stacked-sequence {
                      seq-local: [w409 _ _] -> [_ w431 _]
                      seq-local: [w408 _ _] -> [_ _ w498]
                      seq-local: [w395 _ _] -> [_ _ w499]
                      tunnel: w377 -> [_ w443 w504]
                      tunnel: w378 -> [_ _ w495]
                      tunnel: [_ _ w502] -> w380
                      tunnel: [_ _ w501] -> w376
                      tunnel: w379 -> [_ _ _]
                      tunnel: [w410 _ _] -> w375
                      frame #0 {
                        w391 = T3."Write Element" ("Action")
                        # "SMU data"
                        n224 = Get Date/Time In Seconds() -> (seconds since 1Jan1904=w383:timestamp)
                        n225 = Format Date/Time String(time format string (%c)="%H:%M:%S", seconds (now)=w383) -> (date/time string=w381:string)  [unwired: 1 in]
                        n226 = local write "Last reading at:"(w381) -> ()
                        n227 = local write "STATUS 1"("Reading LCR meter..." ("status")) -> ()
                        n228 = global read "QC_MeasurementSetup.vi" "CV Measurement Parameters"() -> (w407:T8)
                        n229 = Unbundle By Name(w407) -> ("Temperature Readout"=w385:enum16{"Read Arduino", "Enter manually"}, "Arduino"=w384:refnum<class "ArduinoControl.lvclass">, "LCR"=w401:refnum<class "LCRControl.lvclass">, "AC frequency [Hz]"=w386:i32, "Supply"=w402:refnum<class "SupplyControl.lvclass">, "Set Current Limit?"=w406:bool, "Current Limit [µA]"=w404:dbl)
                        n230 = local read "Current reading No."() -> (w390:u32)
                        n231 = case shown="\"Read Arduino\"" w385 {
                          tunnel: [w416 w419] -> w388
                          tunnel: [w413 w422] -> w393
                          tunnel: w384 -> [_ w421]
                          frame "Enter manually", Default {
                            n232 = local read "Temp."() -> (w418:dbl[])
                            n233 = local read "RH"() -> (w414:dbl[])
                            n234 = Index Array(array=w418, index=0) -> (element=w416:dbl)
                            n235 = Index Array(array=w414, index=0) -> (element=w413:dbl)
                          }
                          frame "Read Arduino" {
                            n236 = call "ArduinoRead.vi"("Arduino function"=enum16{"T/RH", "Interlock", "Edgesense"}."T/RH", "ArduinoControl in"=w421) -> ("rel. Humidity [%]"=w422:dbl, "Temperature [°C]"=w419:dbl)  [unwired: 4 in, 4 out]
                          }
                        }
                        n237 = local read "Current Volts:"() -> (w394:dbl)
                        n238 = Multiply(x=w404, y=1000.0) -> (x*y=w403:dbl)
                        n239 = call-dynamic "Supply_ReadCurrent.vi"("SupplyControl in"=w402) -> ("error out"=w396:errorcluster, "Current in nA"=w411:dbl, "SupplyControl out"=w408:refnum<class "SupplyControl.lvclass">)  [unwired: 8 in]
                        n240 = case shown="True" w406 {
                          tunnel: w411 -> [_ w427]
                          tunnel: w403 -> [_ w425]
                          tunnel: [FALSE w424] -> w410
                          frame False {
                          }
                          frame True {
                            n241 = Absolute Value(x=w427) -> (abs(x)=w426:dbl)
                            n242 = Greater?(x=w426, y=w425) -> (0:w424:bool)
                          }
                        }
                        n243 = call "CVData.vi"("Action"=w391, "Array No."=0, "Array Size / Index"=w390, "Data IN"=w394) -> ()  [unwired: 1 in, 2 out]
                        n244 = call-dynamic "LCR_Readout.vi"("error in (no error)"=w396, "Frequency in Hz"=w386, "LCRControl in"=w401) -> ("error out"=w395:errorcluster, "Resistance in Ohm"=w389:dbl, "Capacitance in pF"=w387:dbl)  [unwired: 5 in, 1 out]
                        n245 = Increment(x=w390) -> (x+1=w409:u32)
                        n246 = local write "Current reading No."(w409) -> ()
                        n247 = call "CVData.vi"("Action"=w391, "Array No."=u32 1, "Array Size / Index"=w390, "Data IN"=w387) -> ()  [unwired: 1 in, 2 out]
                        n248 = call "CVData.vi"("Action"=w391, "Array No."=u32 2, "Array Size / Index"=w390, "Data IN"=w389) -> ()  [unwired: 1 in, 2 out]
                        n249 = call "CVData.vi"("Action"=w391, "Array No."=u32 3, "Array Size / Index"=w390, "Data IN"=w388) -> ()  [unwired: 1 in, 2 out]
                        n250 = call "CVData.vi"("Action"=w391, "Array No."=u32 4, "Array Size / Index"=w390, "Data IN"=w393) -> ()  [unwired: 1 in, 2 out]
                      }
                      frame #1 {
                        w440 = u32 5 ("y")
                        # "Update plots"
                        n251 = property on="Cgraph" class="WFGraph (strict)"() -> ("YScale.Mapping Mode"=w432:u8)  [unwired: 2 in, 2 out]
                        n252 = Greater?(x=w431, y=w440) -> (0:w439:bool)
                        n253 = call "CVData.vi"("Action"=T3."Read Array", "Array No."=1) -> ("Array OUT"=w429:dbl[])  [unwired: 3 in, 1 out]
                        n254 = case shown="True" w439 {
                          tunnel: w431 -> [w448 w451]
                          tunnel: w440 -> [_ w450]
                          tunnel: [w448 w450] -> w438
                          tunnel: [0 w449] -> w436
                          frame False {
                          }
                          frame True {
                            n255 = Subtract(x=w451, y=w450) -> (x-y=w449:u32)
                          }
                        }
                        n256 = property on="Cgraph" class="WFGraph (strict)"("YScale.Minimum"=w432) -> ()  [unwired: 2 in, 2 out]
                        n257 = Array Subset(array=w429, index=0, length=w431) -> (w435:dbl[])
                        n258 = local read "Cscale"() -> (w441:enum16{"1/C^2 [1/nF^2]", "nF", "pF"})
                        n259 = Absolute Value(x=w435) -> (abs(x)=w434:dbl[])
                        n260 = case shown="..\"1/C^2 [1/nF^2]\"" w441 {
                          tunnel: [w484 w487 w490] -> w446
                          tunnel: w434 -> [w482 w489 w490]
                          frame .."1/C^2 [1/nF^2]" {
                            n261 = Array Size(array=w482) -> (size(s)=w483:i32)
                            n262 = for {
                              N: w483 -> [_]
                              tunnel: w482 -> [w486] mode=indexing
                              tunnel: [w485] -> w484 mode=indexing
                              n263 = formula code="y=1000000./(x*x);"("x"=w486) -> ("y"=w485:dbl)
                            }
                          }
                          frame "nF" {
                            n264 = Divide(x=w489, y=1000.0) -> (x/y=w487:dbl[])
                          }
                          frame "pF".. {
                          }
                        }
                        n265 = for {
                          N: 5 -> [_]
                          tunnel: w438 -> [w457]
                          tunnel: w436 -> [w456]
                          tunnel: w431 -> [w455]
                          i -> [w453]
                          n266 = call "CVData.vi"("Action"=T3."Read Array", "Array No."=w453) -> ("Array OUT"=w452:dbl[])  [unwired: 3 in, 1 out]
                          n267 = case shown="2" w453 {
                            tunnel: w457 -> [w460 w464 w469 _ _]
                            tunnel: w456 -> [w461 w465 w470 _ _]
                            tunnel: w452 -> [w459 w463 w471 w475 w480]
                            tunnel: w455 -> [_ _ _ w473 w478]
                            frame ..0 {
                              n268 = Array Subset(array=w459, index=w461, length=w460) -> (w458:dbl[])
                              n269 = local write "Volts"(w458) -> ()
                            }
                            frame 1 {
                              n270 = Array Subset(array=w463, index=w465, length=w464) -> (w462:dbl[])
                              n271 = local write "Capacitance"(w462) -> ()
                            }
                            frame 2 {
                              n272 = Array Subset(array=w471, index=w470, length=w469) -> (w468:dbl[])
                              n273 = Multiply(x=w468, y=0.001) -> (x*y=w467:dbl[])
                              n274 = local write "Resistance"(w467) -> ()
                            }
                            frame 3 {
                              n275 = Decrement(x=w473) -> (x-1=w472:u32)
                              n276 = Array Subset(array=w475, index=w472, length=1) -> (w474:dbl[])
                              n277 = local write "Temp."(w474) -> ()
                            }
                            frame 4.. {
                              n278 = Decrement(x=w478) -> (x-1=w477:u32)
                              n279 = Array Subset(array=w480, index=w477, length=1) -> (w479:dbl[])
                              n280 = local write "RH"(w479) -> ()
                            }
                          }
                        }
                        n281 = local read "Initial volts [V]"() -> (w444:dbl)
                        n282 = Absolute Value(x=w443) -> (abs(x)=w442:dbl)
                        n283 = Bundle("Initial volts [V]"=w444, w442, w446) -> (w433:cluster{"Initial volts [V]":dbl, dbl, dbl[]})  [unwired: 1 in]
                        n284 = local write "Cgraph"(w433) -> ()
                      }
                      frame #2 {
                        # "Increment volts and check for end of loop"
                        n285 = local read "positive ramp?"() -> (w500:bool)
                        n286 = local read "Current Volts:"() -> (w496:dbl)
                        n287 = case shown="True" w500 {
                          tunnel: w495 -> [w507 w511]
                          tunnel: w504 -> [w508 w514]
                          tunnel: [w506 w513] -> w491
                          tunnel: [w505 w510] -> w503
                          tunnel: w496 -> [w509 w512]
                          frame False {
                            n288 = Subtract(x=w509, y=w508) -> (x-y=w505:dbl)
                            n289 = Greater Or Equal?(x=w505, y=w507) -> (x >= y?=w506:bool)
                          }
                          frame True {
                            n290 = Add(x=w512, y=w514) -> (x+y=w510:dbl)
                            n291 = Less Or Equal?(x=w510, y=w511) -> (x <= y?=w513:bool)
                          }
                        }
                        n292 = Quotient & Remainder(x=w496, y=w495) -> (x-y*floor(x/y)=w497:dbl, floor(x/y)=w494:dbl)
                        n293 = Not Equal To 0?(x=w497) -> (x != 0?=w492:bool)
                        n294 = Equal To 0?(x=w494) -> (x = 0?=w493:bool)
                        n295 = Or(x=w492, y=w493) -> ()  [unwired: 1 out]
                        n296 = case shown="True" w491 {
                          tunnel: w503 -> [_ w525]
                          tunnel: [TRUE FALSE] -> w502
                          tunnel: [FALSE w526] -> w501
                          tunnel: w496 -> [_ w523]
                          tunnel: w499 -> [_ w522]
                          tunnel: w498 -> [_ w521]
                          frame False {
                          }
                          frame True {
                            n297 = local read "step [V]"() -> (w519:dbl)
                            n298 = call "SupplyRamp.vi"("error in"=w522, "Requested Voltage"=w525, "Step Size"=w519, "Step Delay"=100, "Supply IN"=w521, "Starting Voltage"=w523) -> ("error out"=w517:errorcluster, "Compliance exceeded"=w526:bool, "Current Voltage"=w520:dbl)  [unwired: 2 in, 1 out]
                            n299 = case shown="No Error" w517 {
                              tunnel: w520 -> [w528 _]
                              frame No Error {
                                n300 = local write "Current Volts:"(w528) -> ()
                              }
                              frame Error {
                              }
                            }
                            n301 = property on="Bias On/Off:" class="Bool (strict)"("Blinking"=w526) -> ()  [unwired: 2 in, 2 out]
                            n302 = local write "STATUS 1"("Incrementing volts.") -> ()
                          }
                        }
                      }
                    }
                  }
                  frame True {
                    w529 = FALSE
                  }
                }
              }
            }
            n303 = case shown="True" w286 {
              frame False {
              }
              frame True {
                n304 = property on="Bias On/Off:" class="Bool (strict)"("Blinking"=TRUE) -> ()  [unwired: 2 in, 2 out]
              }
            }
            n305 = Build Array(w288, w286, "abort", w287) -> (w292:bool[])
            n306 = Or Array Elements(Boolean array=w292) -> (logical OR=w298:bool)
            n307 = Not(x=w298) -> (.not. x?=w297:bool)
          }
        }
        frame True {
          w531 = FALSE
          # "compliance was exceeded when first voltage applied."
          # "Flag compliance as reason for end of run"
          n308 = local write "STATUS 1"("Run aborted - compliance exceeded.") -> ()
          n309 = Build Array(w531, TRUE, w531, w531) -> (w532:bool[])
        }
      }
      n310 = Search 1D Array(1D array=w275, element=TRUE) -> (index of element=w273:i32)  [unwired: 1 in]
      n311 = Increment(x=w273) -> (x+1=w272:i32)
      n312 = case shown="..0" w272 {
        tunnel: ["" "Run ended normally" "Compliance exceeded" "Run aborted - by user" "Run aborted - Ilimit exceeded"] -> w267
        frame ..0 {
        }
        frame 1 {
        }
        frame 2 {
          # "Determine reason for end of run."
        }
        frame 3 {
        }
        frame 4.. {
        }
      }
      n313 = global read "QC_RunInformation.vi" "Run info"() -> (w271:T6)
      n314 = Bundle By Name(cluster=w271, "End of Run comment:"=w267) -> (w266:T6)
      n315 = Concatenate Strings(w267, "\r\n", "RAMPING DOWN VOLTS") -> (w270:string)
      n316 = global write "QC_RunInformation.vi" "Run info"(w266) -> ()
      n317 = local write "STATUS 1"(w270) -> ()
    }
    frame #4 {
      # "Ramp down and switch off supply"
      n318 = stacked-sequence {
        frame #0 {
          # "Tie up loose ends. Set volts to zero and switch to standby"
          # "Ramp down volts now"
          n319 = global read "QC_MeasurementSetup.vi" "CV Measurement Parameters"() -> (w543:T8)
          n320 = Unbundle By Name(w543) -> ("Supply"=w540:refnum<class "SupplyControl.lvclass">, "Ramp down steps [V]"=w542:dbl, "Ramp down Interval [s]"=w541:i32, "Measurement switch"=w536:refnum<class "Switching.lvclass">, "Measurement switch used?"=w535:bool)
          n321 = local read "Current Volts:"() -> (w548:dbl)
          n322 = Multiply(x=w541, y=1000) -> (x*y=w545:i32)
          n323 = call "SupplyRamp.vi"("Requested Voltage"=0.0, "Step Size"=w542, "Step Delay"=w545, "Supply IN"=w540, "Starting Voltage"=w548) -> ("error out"=w538:errorcluster, "Supply OUT"=w539:refnum<class "SupplyControl.lvclass">, "Current Voltage"=w546:dbl)  [unwired: 3 in, 1 out]
          n324 = call-dynamic "Supply_Stby.vi"("error in (no error)"=w538, "SupplyControl in"=w539) -> ("error out"=w537:errorcluster)  [unwired: 8 in, 1 out]
          n325 = local write "Current Volts:"(w546) -> ()
          n326 = case shown="True" w535 {
            tunnel: w536 -> [_ w551]
            tunnel: w537 -> [_ w550]
            frame False {
            }
            frame True {
              n327 = call-dynamic "MatrixSwitch.vi"("error in (no error)"=w550, "Action"=T4."Reset", "Switching in"=w551) -> ()  [unwired: 6 in, 3 out]
            }
          }
        }
        frame #1 {
          w556 = 0
          n328 = local write "Bias On/Off:"(FALSE ("Visible")) -> ()
          n329 = local write "Current Volts:"(0.0 ("Current Volts:")) -> ()
          n330 = property on="abort" class="Bool (strict)"("DisabledEnum"=2) -> ()  [unwired: 2 in, 2 out]
          n331 = property on="Quit & Save" class="Bool"("DisabledEnum"=w556) -> ()  [unwired: 2 in, 2 out]
          n332 = property on="quit (no save)" class="Bool"("DisabledEnum"=w556) -> ()  [unwired: 2 in, 2 out]
          n333 = local write "STATUS 1"("Run finished. \nSave data?" ("STATUS 1")) -> ()
        }
        frame #2 {
          n334 = Current VI's Path() -> (path=w558:path)
          n335 = call "SaveJPEG.vi"("Test"="CV", "File Path Control"=w558) -> ()  [unwired: 1 in, 2 out]
        }
      }
    }
    frame #5 {
      # "Loop and await decision on whether to save or junk data"
      # "Display and save data"
      n336 = local read "Scales"() -> (w571:T1)
      n337 = local read "Cscale"() -> (w570:enum16{"1/C^2 [1/nF^2]", "nF", "pF"})
      n338 = while {
        shift-left: w570 -> [w645]
        shift-right: [w644] -> _
        shift-left: w571 -> [w647]
        shift-right: [w646] -> _
        tunnel: [w638] -> w573
        tunnel: ["quit (no save)"] -> w572
        stop <- w643 continue-if-true
        n339 = local read "Scales"() -> (w646:T1)
        n340 = local read "Cscale"() -> (w644:enum16{"1/C^2 [1/nF^2]", "nF", "pF"})
        n341 = Not Equal?(x=w647, y=w646) -> (x != y?=w641:bool)
        n342 = Not Equal?(x=w645, y=w644) -> (x != y?=w640:bool)
        n343 = case shown="True" w641 {
          tunnel: w646 -> [_ w674]
          frame False {
          }
          frame True {
            n344 = case shown="..\"Lin - Lin\"" w674 {
              tunnel: [w675 1 0 w680] -> w673
              tunnel: [w675 0 1 w680] -> w672
              frame .."Lin - Lin" {
                w675 = 0
              }
              frame "Log - Lin" {
              }
              frame "Lin - Log" {
              }
              frame "Log - log".. {
                w680 = 1
              }
            }
            n345 = property on="Cgraph" class="WFGraph (strict)"("X Scale.Mapping Mode"=w673) -> ()  [unwired: 2 in, 2 out]
            n346 = property on="Cgraph" class="WFGraph (strict)"("Y Scale.Mapping Mode"=w672, "YScale.Minimum"=w672) -> ()  [unwired: 2 in, 2 out]
          }
        }
        n347 = case shown="True" w640 {
          tunnel: w644 -> [_ w652]
          frame False {
          }
          frame True {
            n348 = property on="Cgraph" class="WFGraph (strict)"() -> ("YScale.Mapping Mode"=w655:u8)  [unwired: 2 in, 2 out]
            n349 = global read "QC_MeasurementSetup.vi" "CV Measurement Parameters"() -> (w654:T8)
            n350 = property on="Cgraph" class="WFGraph (strict)"("YScale.Minimum"=w655) -> ()  [unwired: 2 in, 2 out]
            n351 = Unbundle By Name(w654) -> ("Initial Voltage [V]"=w657:dbl, "Step Size [V]"=w659:dbl, "Number Of Steps"=w656:u32)
            n352 = call "CVData.vi"("Action"=T3."Read Array", "Array No."=u32 1 ("Action")) -> ("Array OUT"=w648:dbl[])  [unwired: 3 in, 1 out]
            n353 = Absolute Value(x=w659) -> (abs(x)=w658:dbl)
            n354 = Array Subset(array=w648, index=0, length=w656) -> (w660:dbl[])
            n355 = Absolute Value(x=w660) -> (abs(x)=w653:dbl[])
            n356 = case shown="..\"1/C^2 [1/nF^2]\"" w652 {
              tunnel: [w665 w668 w671] -> w651
              tunnel: w653 -> [w663 w670 w671]
              frame .."1/C^2 [1/nF^2]" {
                n357 = Array Size(array=w663) -> (size(s)=w664:i32)
                n358 = for {
                  N: w664 -> [_]
                  tunnel: w663 -> [w667] mode=indexing
                  tunnel: [w666] -> w665 mode=indexing
                  n359 = formula code="y=1000000./(x*x);"("x"=w667) -> ("y"=w666:dbl)
                }
              }
              frame "nF" {
                n360 = Divide(x=w670, y=1000.0) -> (x/y=w668:dbl[])
              }
              frame "pF".. {
              }
            }
            n361 = Bundle("Initial Voltage [V]"=w657, w658, w651) -> (w661:cluster{"Initial Voltage [V]":dbl, dbl, dbl[]})  [unwired: 1 in]
            n362 = local write "Cgraph"(w661) -> ()
          }
        }
        n363 = local read "Run uninterrupted?"() -> (w637:bool)
        n364 = Or(x=w637, y="Auto save files") -> (x .or. y?=w635:bool)
        n365 = Select(t=w635, s=w635, f="Quit & Save") -> (s? t:f=w638:bool)
        n366 = Not Or(1:"quit (no save)", 2:w638) -> (0:w643:bool)
      }
      n367 = global read "QC_MeasurementSetup.vi" "CV Measurement Parameters"() -> (w569:T8)
      n368 = Unbundle By Name(w569) -> ("Temperature Readout"=w568:enum16{"Read Arduino", "Enter manually"}, "Arduino"=w562:refnum<class "ArduinoControl.lvclass">)
      n369 = case shown="\"Read Arduino\"" w568 {
        tunnel: w562 -> [_ w634]
        frame "Enter manually", Default {
        }
        frame "Read Arduino" {
          n370 = call "ArduinoClose.vi"("ArduinoControl in"=w634) -> ()  [unwired: 9 in, 2 out]
        }
      }
      n371 = case shown="True" w572 {
        tunnel: [FALSE w682] -> w574
        frame False {
        }
        frame True {
          n372 = Two Button Dialog(message="Are you sure you don't want to save the data?", 1:"Quit" ("F button name (\"Cancel\")"), 2:"Save data" ("T button name (\"OK\")")) -> (T button?=w682:bool)
        }
      }
      n373 = Or(x=w573, y=w574) -> (x .or. y?=w567:bool)
      n374 = flat-sequence {
        tunnel: w567 -> [w586]
        tunnel: [w586] -> w560
        tunnel: [TRUE] -> w559
        tunnel: [w632] -> w561
        tunnel: [w633] -> w563
        tunnel: w560 -> [w633]
        tunnel: w559 -> [w632]
        frame #0 {
          n375 = global read "QC_MeasurementSetup.vi" "CV Measurement Parameters"() -> (w595:T8)
          n376 = Unbundle By Name(w595) -> ("V_depletion Limit [V]"=w588:dbl)
          n377 = call "ScanFeedback.vi"("measurement type"=T5."CV") -> ("V depletion"=w590:dbl)  [unwired: 4 in, 4 out]
          n378 = Absolute Value(x=w590) -> (abs(x)=w589:dbl)
          n379 = Absolute Value(x=w588) -> (abs(x)=w587:dbl)
          n380 = Less Or Equal?(x=w589, y=w587) -> (x <= y?=w591:bool)
          n381 = local read "Run uninterrupted?"() -> (w584:bool)
          n382 = local read "Auto save files"() -> (w583:bool)
          n383 = Or(x=w584, y=w583) -> (x .or. y?=w575:bool)
          n384 = case shown="True" w586 {
            tunnel: ["" w630] -> w596
            tunnel: [_ w617] -> w594
            tunnel: [_ w599] -> w579
            tunnel: w575 -> [_ w598]
            frame False {
            }
            frame True {
              w615 = T3."Read Array" ("Action")
              n385 = local write "STATUS 1"("Saving Data ...") -> ()
              n386 = call "CVData.vi"("Action"=w615, "Array No."=u32 2 ("Action")) -> ("Array OUT"=w613:dbl[])  [unwired: 3 in, 1 out]
              n387 = Multiply(x=w613, y=1e-06) -> (x*y=w612:dbl[])
              n388 = call "CVData.vi"("Action"=w615, "Array No."=u32 0 ("Action")) -> ("Array OUT"=w621:dbl[])  [unwired: 3 in, 1 out]
              n389 = call "CVData.vi"("Action"=w615, "Array No."=u32 1 ("Action")) -> ("Array OUT"=w620:dbl[])  [unwired: 3 in, 1 out]
              n390 = Build Array(w621, w620, w612) -> (w619:dbl[][])
              n391 = call "CVData.vi"("Action"=w615, "Array No."=u32 4 ("Action")) -> ("Array OUT"=w627:dbl[])  [unwired: 3 in, 1 out]
              n392 = call "CVData.vi"("Action"=w615, "Array No."=u32 3 ("Action")) -> ("Array OUT"=w626:dbl[])  [unwired: 3 in, 1 out]
              n393 = local read "Current reading No."() -> (w607:u32)
              n394 = Add Array Elements(numeric array=w627) -> (sum=w610:dbl)
              n395 = Add Array Elements(numeric array=w626) -> (sum=w608:dbl)
              n396 = Transpose 2D Array(2D array=w619) -> (transposed array=w602:dbl[][])
              n397 = Array Size(array=w602) -> (size(s)=w605:i32[])
              n398 = Divide(x=w608, y=w607) -> (x/y=w606:dbl)
              n399 = Divide(x=w610, y=w607) -> (x/y=w609:dbl)
              n400 = Index Array(array=w605, index #1=0, index #2=1) -> (element #1=w601:i32, element #2=w600:i32)
              n401 = call "SaveDataFile.vi"("Data Array"=w602, "Temperature"=w606, "Run uninterrupted?"=w598, "Humidity"=w609, "no. of arrays"=w600, "Actual array lengths"=w601, "Array Titles"="Voltage[V] Capacitance[pF] Resistance[MOhm]", "Strip Segment"="", "Arrays format"="%010.2f") -> ("Filename OUT"=w599:string, "Path + Filename OUT"=w630:string, "Error Out"=w617:errorcluster)  [unwired: 3 in, 1 out]
            }
          }
          n402 = global read "QC_RunInformation.vi" "LocalConfiguration"() -> (w577:T7)
          n403 = call "WriteLogFile.vi"("Run uninterrupted?"=w575, "Automatic warning"="", "Data File"=w596, "Error In"=w594, "DUT passed?"=w591, "Value TechSpec criteria"=w590, "Files saved?"=w586) -> ()  [unwired: 4 in, 1 out]
          n404 = Unbundle By Name(w577) -> ("Backup & screenshot directory"=w576:string)
          n405 = Search/Split String(string=w579, search string/char (-)=".dat") -> (substring before match=w578:string)  [unwired: 1 in, 2 out]
          n406 = String To Path(string=w576) -> (path=w582:path)
          n407 = control-ref of="This VI"() -> (w581:refnum<vi>)
          n408 = call "CreateScreenShot.vi"("Screenshot name"=w578, "base path"=w582, "reference"=w581) -> ()  [unwired: 8 in, 1 out]
        }
        frame #1 {
          w631 = FALSE
          n409 = local write "Run uninterrupted?"(w631) -> ()
          n410 = local write "Wait for continue"(w631) -> ()
        }
      }
      n411 = Select(t="Run finished.\nData saved." ("STATUS 1"), s=w563, f="Run finished.\nData not saved." ("STATUS 1")) -> (s? t:f=w566:string)
      n412 = local write "STATUS 1"(w566) -> ()
      "Done!" <- w561
    }
  }
